vi "numElements.vi"(8 "error in (no error)":errorcluster, 11 "InconsistentList in":refnum<class "NI_Robotics_InconsistentList.lvclass">) -> (0 "error out":errorcluster, 2 "number of list elements":i32, 3 "InconsistentList out":refnum<class "NI_Robotics_InconsistentList.lvclass">)   [LabVIEW 2017, in "NI_Robotics_InconsistentList.lvclass"]
uses:
  <vilib>/robotics/Navigation/shared/InconsistentList/NI_Robotics_InconsistentList.lvclass
  <vilib>/robotics/Navigation/shared/InconsistentList/NI_Robotics_InconsistentList.lvclass/NI_Robotics_InconsistentList.ctl
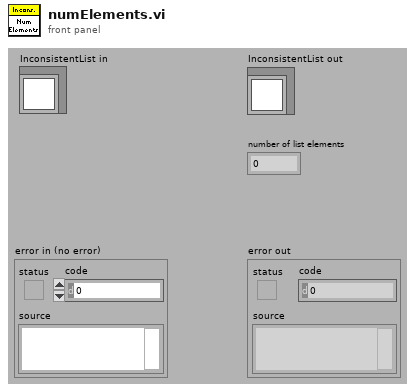
[diagram p1: front panel]
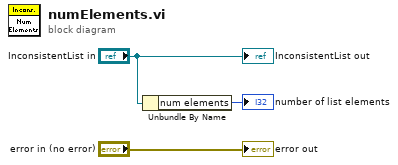
[diagram p0: block diagram]
diagram:
  n1 = Unbundle By Name("InconsistentList in") -> ("num elements"=→"number of list elements":i32)
  "InconsistentList out" <- "InconsistentList in"
  "error out" <- "error in (no error)"
